vi "Keyence LJ-X8000A Read Profile Data.vi"() -> ()   [LabVIEW 2010]
doc: "This example mainly indicates how to acquire profiles from controllers \nby using <B>Read Profile Array</B> and <B>Read Batch Profile All</B> VIs."
uses:
  KEYENCE LJ-X8000A.lvlib
  Public/Clusters/Ethernet Config.ctl
  Public/Clusters/Profile Info.ctl
  Public/Clusters/Read Profile Rsp.ctl
  Public/Constants/Profile Pos.ctl
  Public/Clusters/Read Profile Req.ctl
  Public/Clusters/Read Batch Profile Rsp.ctl
  Public/Constants/Batch Pos.ctl
panel:
  in  "tab1":T1(tab)
  out "Height Profile":T2(graph)
  out "Profile Info":T3
  out "Profile Rsp":T4
  out "Brightness Profile":T5(graph)
  in  "Read Req":T6={"Read Area"=enum."ACTIVE_BANK", "Profile Pos"=0, "Read Profile No."=0, "Read Profile Cnt"=1, "isErase"=FALSE} {"Profile Pos" items=["CURRENT", "OLDEST", "SPECIFY"]}
  in  "btnStartMonitoring":bool
  in  "btnStopMonitoring":bool
  out "isConnecting":bool caption="Monitoring"
  out "error out":errorcluster {"code" format="%.0x"}
  out "read status":u8(slide) scale=0.0..100.0
  in  "btnReadBatchProfiles":bool
  in  "btnBatchStop":bool
  in  "btnBatchStart":bool
  out "isBatchReading":bool caption="Reading"
  out "Batch Height Image":dbl[][](graph)
  in  "Read Batch Profile Req":T9 {"Batch Pos" items=["CURRENT"=0, "SPECIFY"=2, "COMMITED"=3, "NEWEST PROFILE"=4]}
  in  "Read Profile Cnt":u32=1000
  out "Batch Profile Info":T3
  out "Read Batch Profile Rsp":T10
  in  "Timeout(ms)":u32=5000
  out "error out 2":errorcluster caption="error out" {"code" format="%.0x"}
  out "Timeout ?":bool
  in  "Ethernet Config":T11={"IP Address"=[192, 168, 0, 1], "Port No"=24691}
  in  "stop":bool caption="’âŽ~"
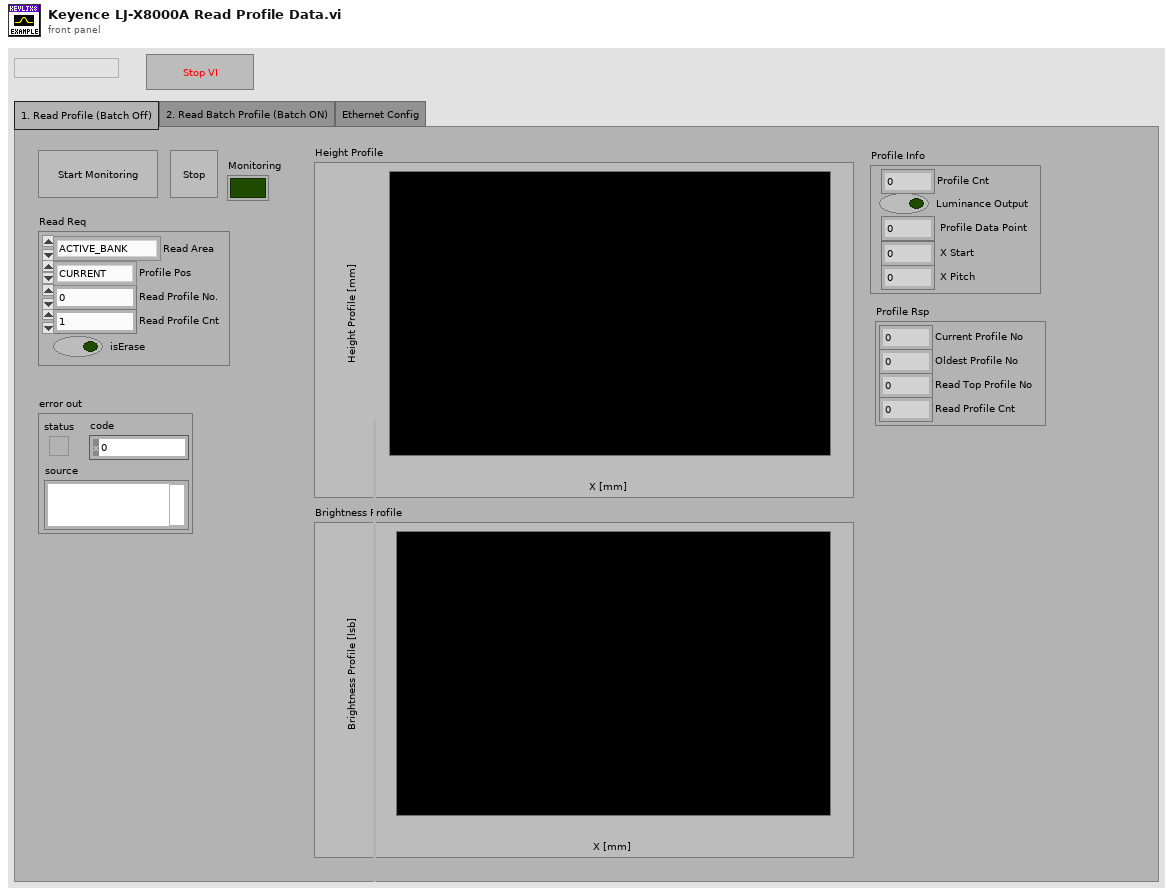
[diagram p1: front panel]
types:
  T1 = enum32{"1. Read Profile (Batch Off)", "2. Read Batch Profile (Batch ON)", "Ethernet Config"}
  T2 = cluster{" X Start":dbl, " X Pitch":dbl, "Height Profile Array":dbl[]}
  T3 = typedef "KEYENCE LJ-X8000A.lvlib/Profile Info.ctl" = cluster{"Profile Cnt":u8, "Luminance Output":bool, " Profile Data Point":u16, " X Start":i32, " X Pitch":i32}
  T4 = typedef "KEYENCE LJ-X8000A.lvlib/Read Profile Rsp.ctl" = cluster{"Current Profile No":u32, "Oldest Profile No":u32, "Read Top Profile No":u32, "Read Profile Cnt":u8}
  T5 = cluster{" X Start":dbl, " X Pitch":dbl, "Luminance Profile Array":u16[]}
  T6 = typedef "KEYENCE LJ-X8000A.lvlib/Read Profile Req.ctl" = cluster{"Read Area":enum8{"ACTIVE_BANK", "INACTIVE_BANK"}, "Profile Pos":T7, "Read Profile No.":u32, "Read Profile Cnt":u8, "isErase":bool}
  T7 = typedef "KEYENCE LJ-X8000A.lvlib/Profile Pos.ctl" = u8
  T8 = typedef "KEYENCE LJ-X8000A.lvlib/Batch Pos.ctl" = u8
  T9 = cluster{"Read Area":enum8{"ACTIVE_BANK", "INACTIVE_BANK"}, "Batch Pos":T8, "Read Batch No":u32, "isErase":bool}
  T10 = typedef "KEYENCE LJ-X8000A.lvlib/Read Batch Profile Rsp.ctl" = cluster{"Current Batch No":u32, "Current Batch Profile Cnt":u32, "Oldest Batch No":u32, "Oldest Batch Profile Cnt":u32, "Read Batch No":u32, "Read Batch Profile Cnt":u32, "Read Batch Top Profile No":u32, "Read Profile Cnt":u32, "Current Batch Commited":bool}
  T11 = typedef "KEYENCE LJ-X8000A.lvlib/Ethernet Config.ctl" = cluster{"IP Address":u8[], "Port No":u16}
  T12 = enum8{"Enabled", "Disabled", "Disabled and Grayed Out"}
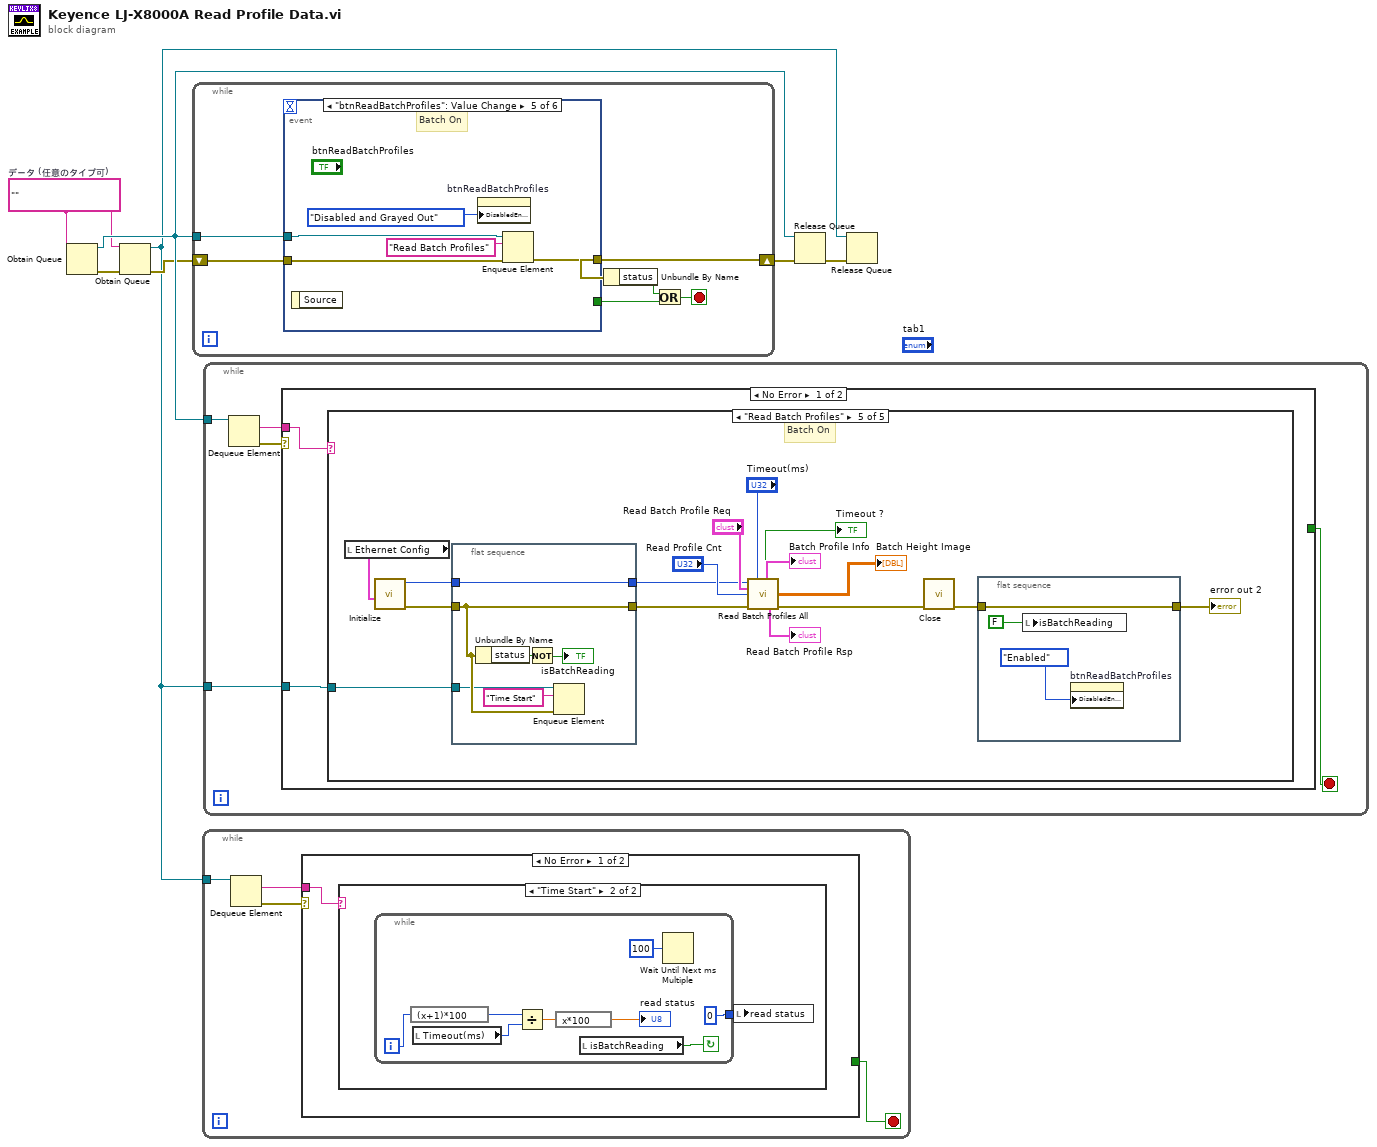
[diagram p0: block diagram]
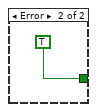
[diagram p3: hidden frame]
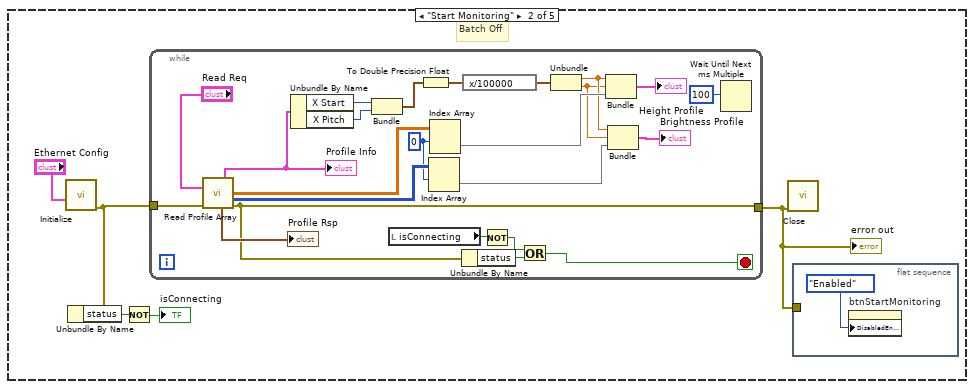
[diagram p5: hidden frame]
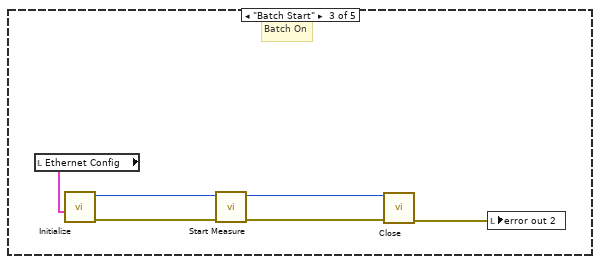
[diagram p6: hidden frame]
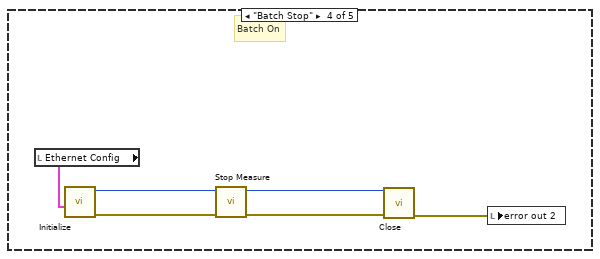
[diagram p7: hidden frame]
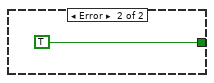
[diagram p8: hidden frame]
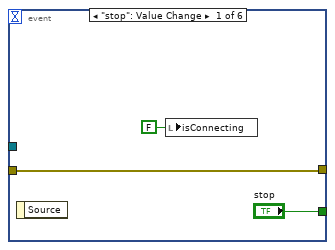
[diagram p9: hidden frame]
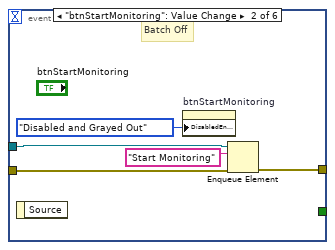
[diagram p10: hidden frame]
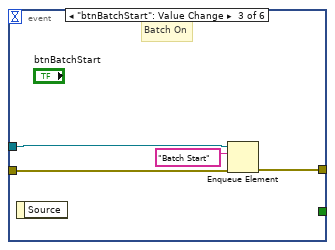
[diagram p11: hidden frame]
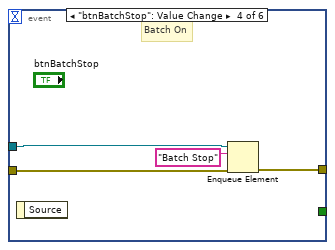
[diagram p12: hidden frame]
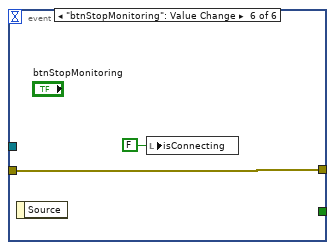
[diagram p13: hidden frame]
diagram:
  w3 = ""  # データ (任意のタイプ可)
  n1 = Obtain Queue(element data type=w3) -> (queue out=w6:refnum<queue>, error out=w5:errorcluster)  [unwired: 4 in, 1 out]
  n2 = Obtain Queue(element data type=w3, error in (no error)=w5) -> (queue out=w1:refnum<queue>, error out=w4:errorcluster)  [unwired: 3 in, 1 out]
  n3 = while {
    shift-right: [w9] -> w7
    shift-left: w4 -> [w12]
    tunnel: w6 -> [w13]
    stop <- w10 stop-if-true
    n4 = event shown="[4] \"btnReadBatchProfiles\": Value Change" {
      selector: _ -> [_ _ _ _ _ _]
      dyn-events: _ -> [_ _ _ _ _ _]
      timeout: _ -> [_ _ _ _ _ _]
      tunnel: w13 -> [_ w18 w22 w26 w31 _]
      tunnel: w12 -> [w15 w19 w23 w27 w32 w36]
      tunnel: [w15 w20 w24 w28 w33 w36] -> w9
      tunnel: ["stop" _ _ _ _ _] -> w11
      event "stop": Value Change {
        n5 = event-data() -> ()  [unwired: 1 in, 1 out]
        n6 = local write "isConnecting"(FALSE ("isConnecting")) -> ()
      }
      event "btnStartMonitoring": Value Change {
        # "Batch Off"
        n7 = event-data() -> ()  [unwired: 1 in, 1 out]
        n8 = property on="btnStartMonitoring" class="Bool"("DisabledEnum"=T12."Disabled and Grayed Out" ("–³Œø")) -> ()  [unwired: 2 in, 2 out]
        n9 = Enqueue Element(queue=w18, element="Start Monitoring", error in (no error)=w19) -> (error out=w20:errorcluster)  [unwired: 1 in, 2 out]
      }
      event "btnBatchStart": Value Change {
        # "Batch On"
        n10 = event-data() -> ()  [unwired: 1 in, 1 out]
        n11 = Enqueue Element(queue=w22, element="Batch Start", error in (no error)=w23) -> (error out=w24:errorcluster)  [unwired: 1 in, 2 out]
      }
      event "btnBatchStop": Value Change {
        # "Batch On"
        n12 = event-data() -> ()  [unwired: 1 in, 1 out]
        n13 = Enqueue Element(queue=w26, element="Batch Stop", error in (no error)=w27) -> (error out=w28:errorcluster)  [unwired: 1 in, 2 out]
      }
      event "btnReadBatchProfiles": Value Change {
        # "Batch On"
        n14 = event-data() -> ()  [unwired: 1 in, 1 out]
        n15 = property on="btnReadBatchProfiles" class="Bool"("DisabledEnum"=T12."Disabled and Grayed Out" ("–³Œø")) -> ()  [unwired: 2 in, 2 out]
        n16 = Enqueue Element(queue=w31, element="Read Batch Profiles", error in (no error)=w32) -> (error out=w33:errorcluster)  [unwired: 1 in, 2 out]
      }
      event "btnStopMonitoring": Value Change {
        n17 = event-data() -> ()  [unwired: 1 in, 1 out]
        n18 = local write "isConnecting"(FALSE ("isConnecting")) -> ()
      }
    }
    n19 = Unbundle By Name(w9) -> ("status"=w8:bool)
    n20 = Or(x=w8, y=w11) -> (x .or. y?=w10:bool)
  }
  n21 = while {
    tunnel: w1 -> [w40]
    stop <- w37 stop-if-true
    n22 = Dequeue Element(queue=w40) -> (element=w38:string, error out=w39:errorcluster)  [unwired: 2 in, 2 out]
    n23 = case shown="No Error" w39 {
      tunnel: w38 -> [w41 _]
      tunnel: [_ TRUE] -> w37
      frame No Error {
        n24 = case shown="\"Time Start\"" w41 {
          frame "FALSE", Default {
          }
          frame "Time Start" {
            n25 = while {
              tunnel: [u32 0 ("ミリ秒倍数")] -> w42
              i -> [w49]
              stop <- w44 continue-if-true
              n26 = expression code="(x+1)*100"(w49) -> (w48:i32)
              n27 = local read "Timeout(ms)"() -> (w47:u32)
              n28 = Divide(x=w48, y=w47) -> (x/y=w46:dbl)
              n29 = expression code="x*100"(w46) -> (→"read status":dbl)
              n30 = local read "isBatchReading"() -> (w44:bool)
              n31 = Wait Until Next ms Multiple(millisecond multiple=u32 100 ("ミリ秒倍数")) -> ()  [unwired: 1 out]
            }
            n32 = local write "read status"(w42) -> ()
          }
        }
      }
      frame Error {
      }
    }
  }
  n33 = while {
    tunnel: w6 -> [w56]
    tunnel: w1 -> [w52]
    stop <- w53 stop-if-true
    n34 = Dequeue Element(queue=w56) -> (element=w54:string, error out=w55:errorcluster)  [unwired: 2 in, 2 out]
    n35 = case shown="No Error" w55 {
      tunnel: w54 -> [w58 _]
      tunnel: [_ TRUE] -> w53
      tunnel: w52 -> [w57 _]
      frame No Error {
        n36 = case shown="\"Read Batch Profiles\"" w58 {
          tunnel: w57 -> [_ _ _ _ w102]
          frame "FALSE", Default {
          }
          frame "Start Monitoring" {
            # "Batch Off"
            n37 = call "Initialize.vi"("Ethernet Config"="Ethernet Config") -> ("error out"=w61:errorcluster)  [unwired: 9 in, 1 out]
            n38 = Unbundle By Name(w61) -> ("status"=w62:bool)
            n39 = Not(x=w62) -> (.not. x?=→"isConnecting":bool)
            n40 = while {
              tunnel: w61 -> [w88]
              tunnel: [w82] -> w59
              stop <- w87 stop-if-true
              w70 = 0 ("wW (s)")
              n41 = call "Read Profile Array.vi"("Read Req"="Read Req", "error in (no error)"=w88) -> ("Profile Info"=w80:T3, "Height Profile Array"=w81:dbl[][], "Luminance Profile Array"=w71:u16[][], "Profile Rsp"=→"Profile Rsp":T4, "error out"=w82:errorcluster)  [unwired: 7 in, 2 out]
              "Profile Info" <- w80
              n42 = Unbundle By Name(w80) -> ("X Start"=w79:i32, "X Pitch"=w78:i32)
              n43 = Bundle("X Start"=w79, "X Pitch"=w78) -> (w77:cluster{" X Start":i32, " X Pitch":i32})  [unwired: 1 in]
              n44 = local read "isConnecting"() -> (w84:bool)
              n45 = To Double Precision Float(number=w77) -> (double precision float=w76:cluster{" X Start":dbl, " X Pitch":dbl})
              n46 = Index Array(array=w71, index (row)=w70) -> (element=w69:u16[])  [unwired: 1 in]
              n47 = Index Array(array=w81, index (row)=w70) -> (element=w74:dbl[])  [unwired: 1 in]
              n48 = Unbundle By Name(w82) -> ("status"=w65:bool)
              n49 = expression code="x/100000"(w76) -> (w75:cluster{" X Start":dbl, " X Pitch":dbl})
              n50 = Not(x=w84) -> (.not. x?=w83:bool)
              n51 = Or(x=w83, y=w65) -> (x .or. y?=w87:bool)
              n52 = Unbundle(w75) -> ("X Start"=w73:dbl, "X Pitch"=w72:dbl)
              n53 = Bundle("X Start"=w73, "X Pitch"=w72, "Height Profile Array"=w74) -> (→"Height Profile":T2)  [unwired: 1 in]
              n54 = Bundle("X Start"=w73, "X Pitch"=w72, "Luminance Profile Array"=w69) -> (→"Brightness Profile":T5)  [unwired: 1 in]
              n55 = Wait Until Next ms Multiple(millisecond multiple=u32 100 ("ミリ秒倍数")) -> ()  [unwired: 1 out]
            }
            "error out" <- w59
            n56 = call "Close.vi"("error in (no error)"=w59) -> ()  [unwired: 9 in, 2 out]
            n57 = flat-sequence {
              tunnel: w59 -> [_]
              frame #0 {
                n58 = property on="btnStartMonitoring" class="Bool"("DisabledEnum"=T12."Enabled" ("–³Œø")) -> ()  [unwired: 2 in, 2 out]
              }
            }
          }
          frame "Batch Start" {
            # "Batch On"
            n59 = local read "Ethernet Config"() -> (w94:T11)
            n60 = call "Initialize.vi"("Ethernet Config"=w94) -> ("error out"=w93:errorcluster, "Device ID out"=w92:i32)  [unwired: 9 in]
            n61 = call "Start Measure.vi"("error in (no error)"=w93, "Device ID (0)"=w92) -> ("error out"=w91:errorcluster, "Device ID out"=w90:i32)  [unwired: 8 in]
            n62 = call "Close.vi"("error in (no error)"=w91, "Device ID (0)"=w90) -> ("error out"=w89:errorcluster)  [unwired: 8 in, 1 out]
            n63 = local write "error out 2"(w89) -> ()
          }
          frame "Batch Stop" {
            # "Batch On"
            n64 = local read "Ethernet Config"() -> (w100:T11)
            n65 = call "Initialize.vi"("Ethernet Config"=w100) -> ("error out"=w99:errorcluster, "Device ID out"=w98:i32)  [unwired: 9 in]
            n66 = call "Stop Measure.vi"("error in (no error)"=w99, "Device ID (0)"=w98) -> ("error out"=w97:errorcluster, "Device ID out"=w96:i32)  [unwired: 8 in]
            n67 = call "Close.vi"("error in (no error)"=w97, "Device ID (0)"=w96) -> ("error out"=w95:errorcluster)  [unwired: 8 in, 1 out]
            n68 = local write "error out 2"(w95) -> ()
          }
          frame "Read Batch Profiles" {
            # "Batch On"
            n69 = local read "Ethernet Config"() -> (w116:T11)
            n70 = call "Initialize.vi"("Ethernet Config"=w116) -> ("error out"=w104:errorcluster, "Device ID out"=w106:i32)  [unwired: 9 in]
            n71 = flat-sequence {
              tunnel: w106 -> [w122]
              tunnel: [w122] -> w105
              tunnel: w104 -> [w119]
              tunnel: [w119] -> w103
              tunnel: w102 -> [w118]
              frame #0 {
                n72 = Unbundle By Name(w119) -> ("status"=w121:bool)
                n73 = Not(x=w121) -> (.not. x?=→"isBatchReading":bool)
                n74 = Enqueue Element(queue=w118, element="Time Start", error in (no error)=w119) -> ()  [unwired: 1 in, 3 out]
              }
            }
            n75 = call "Read Batch Profiles All.vi"("Device ID (0)"=w105, "Timeout ms (5000)"="Timeout(ms)", "Read Batch Profile Req"="Read Batch Profile Req", "Read Profile Cnt"="Read Profile Cnt", "error in (no error)"=w103) -> ("Timeout ?"=→"Timeout ?":bool, "Profile Info"=→"Batch Profile Info":T3, "Height Profile Array"=→"Batch Height Image":dbl[][], "Read Batch Profile Rsp"=→"Read Batch Profile Rsp":T10, "error out"=w109:errorcluster)  [unwired: 3 in, 3 out]
            n76 = call "Close.vi"("error in (no error)"=w109) -> ("error out"=w108:errorcluster)  [unwired: 9 in, 1 out]
            n77 = flat-sequence {
              tunnel: w108 -> [w124]
              tunnel: [w124] -> w107
              frame #0 {
                n78 = local write "isBatchReading"(FALSE ("isBatchMeasureing")) -> ()
                n79 = property on="btnReadBatchProfiles" class="Bool"("DisabledEnum"=T12."Enabled" ("–³Œø")) -> ()  [unwired: 2 in, 2 out]
              }
            }
            "error out 2" <- w107
          }
        }
      }
      frame Error {
      }
    }
  }
  n80 = Release Queue(queue=w6, error in (no error)=w7) -> (error out=w2:errorcluster)  [unwired: 1 in, 2 out]
  n81 = Release Queue(queue=w1, error in (no error)=w2) -> ()  [unwired: 1 in, 3 out]
